vi "Retest check.vi"(0 "SerialNumber":string, 1 "Variant":string) -> (12 "Number of passes":u8, 13 "Number of Fails":u8, 16 "Error Code":i16, 17 "Already passed":bool, 18 "Max Test":bool)   [LabVIEW 2025]
uses:
  <vilib>/Utility/file.llb/Read Delimited Spreadsheet (I64).vi
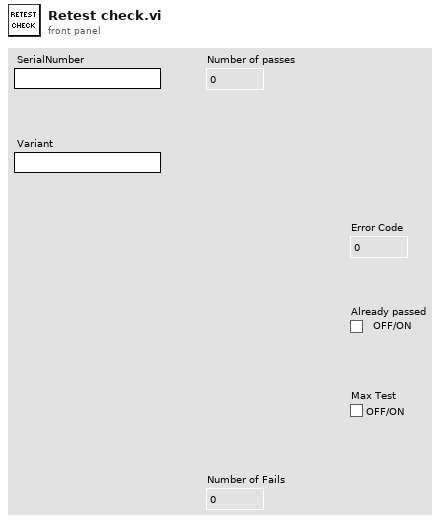
[diagram p1: front panel]
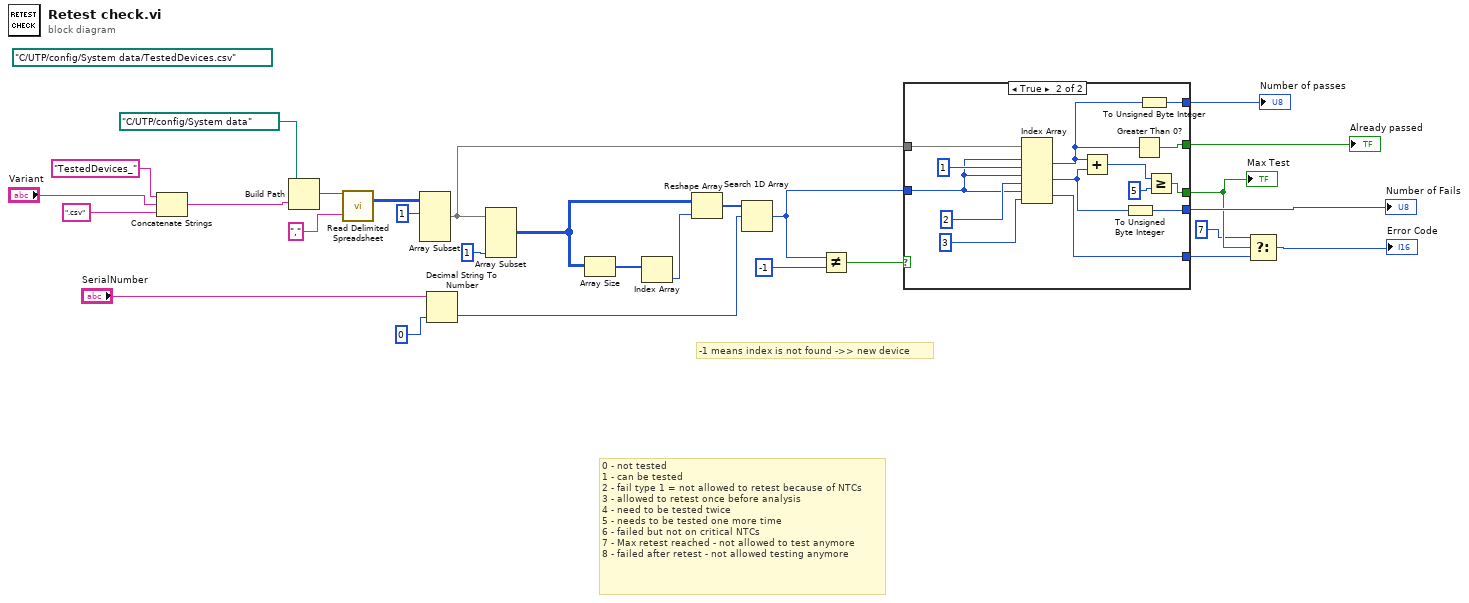
[diagram p0: block diagram]
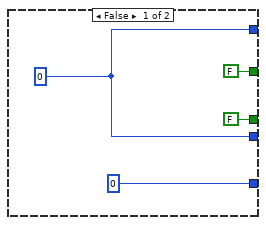
[diagram p2: hidden frame]
diagram:
  (unwired) path "C:/UTP/config/System data/TestedDevices.csv" ("file path (dialog if empty)")
  # "-1 means index is not found ->> new device"
  # "0 - not tested\n1 - can be tested\n2 - fail type 1 = not allowed to retest because of NTCs\n3 - allowed to retest once before analysis\n4 - need to be tested twice\n5 - needs to be tested one more time\n6 - failed but not on critical NTCs\n7 - Max retest reached - not allowed to test anymore\n8 - failed after retest - not allowed testing anymore"
  n1 = Concatenate Strings("TestedDevices_" ("string"), "Variant", ".csv" ("string")) -> (w8:string)
  n2 = Build Path(base path=path "C:/UTP/config/System data" ("file path (dialog if empty)"), name or relative path=w8) -> (appended path=w7:path)
  n3 = call-poly <vilib>:"Read Delimited Spreadsheet.vi"("file path (dialog if empty)"=w7, "delimiter (\\t)"="," ("delimiter (\\t)")) -> ("all rows"=w18:i64[][])  [unwired: 8 in, 5 out]
  n4 = Array Subset(array=w18, index (row)=1 ("index")) -> (w5:i64[][])  [unwired: 3 in]
  n5 = Decimal String To Number(string="SerialNumber", default (0L)=i64 0 ("default (0 I32)")) -> (number=w16:i64)  [unwired: 1 in, 1 out]
  n6 = Array Subset(array=w5, length (col)=1 ("length")) -> (w25:i64[][])  [unwired: 3 in]
  n7 = Array Size(array=w25) -> (size(s)=w24:i32[])
  n8 = Index Array(array=w24) -> (element=w23:i32)  [unwired: 1 in]
  n9 = Reshape Array(w25, w23) -> (w21:i64[])
  n10 = Search 1D Array(1D array=w21, element=w16) -> (index of element=w20:i32)  [unwired: 1 in]
  n11 = Not Equal?(x=w20, y=-1) -> (x != y?=w28:bool)
  n12 = case shown="True" w28 {
    tunnel: w5 -> [_ w46]
    tunnel: w20 -> [_ w38]
    tunnel: [FALSE w42] -> w19
    tunnel: [FALSE w41] -> w4
    tunnel: [w30 w40] -> w14
    tunnel: [w30 w39] -> w13
    tunnel: [i64 0 ("Numeric") w36] -> w3
    frame False {
      w30 = u8 0 ("Numeric")
    }
    frame True {
      n13 = Index Array(array=w46, index (row) #1=w38, index (col) #1=1 ("index (col)"), index (row) #2=w38, index (col) #2=2 ("index (col)"), index (row) #3=w38, index (col) #3=3 ("index (col)")) -> (element #1=w35:i64, element #2=w34:i64, element #3=w36:i64)
      n14 = Add(x=w35, y=w34) -> (x+y=w33:i64)
      n15 = To Unsigned Byte Integer(number=w34) -> (unsigned 8bit integer=w39:u8)
      n16 = Greater Than 0?(x=w35) -> (x > 0?=w42:bool)
      n17 = To Unsigned Byte Integer(number=w35) -> (unsigned 8bit integer=w40:u8)
      n18 = Greater Or Equal?(x=w33, y=i64 5) -> (x >= y?=w41:bool)
    }
  }
  "Already passed" <- w19
  "Max Test" <- w4
  "Number of passes" <- w14
  "Number of Fails" <- w13
  n19 = Select(t=i64 7, s=w4, f=w3) -> (s? t:f=→"Error Code":i64)
